vi "ProjectDataTransToStringForLog.vi"(7 "Class Name":string, 9 "NewVal":variant, 10 "OldVal":variant, 11 "Label.Text":string) -> (1 "NewData":string, 2 "OldData":string, 3 "DataName":string)   [LabVIEW 2019]
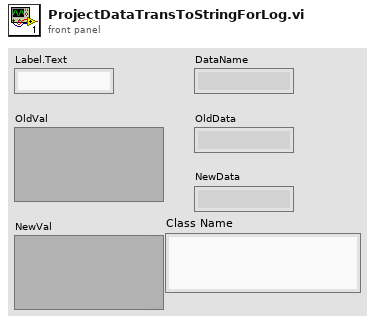
[diagram p1: front panel]
types:
  T1 = cluster{"Yield¢İvertake":dbl, "Fail¢İvertake":dbl, "TestTimeout":sgl, "TrayIn_Retry":dbl, "TrayOut_Retry":dbl, "Errcont":dbl, "back1":dbl, "back2":dbl}
  T2 = cluster{"Yield¢İvertake":dbl, "Fail¢İvertake":dbl, "TestTimeout":dbl, "TrayIn_Retry":dbl, "TrayOut_Retry":dbl, "Errcont":dbl, "back1":dbl, "back2":dbl}
  T3 = cluster{"PC-ID":string, "StationAddress":string}[]
  T4 = cluster{"SHB1":string, "SHB2":string, "SHB3":string, "SHB4":string, "SHB5":string, "SHB6":string, "SHB7":string, "SHB8":string}
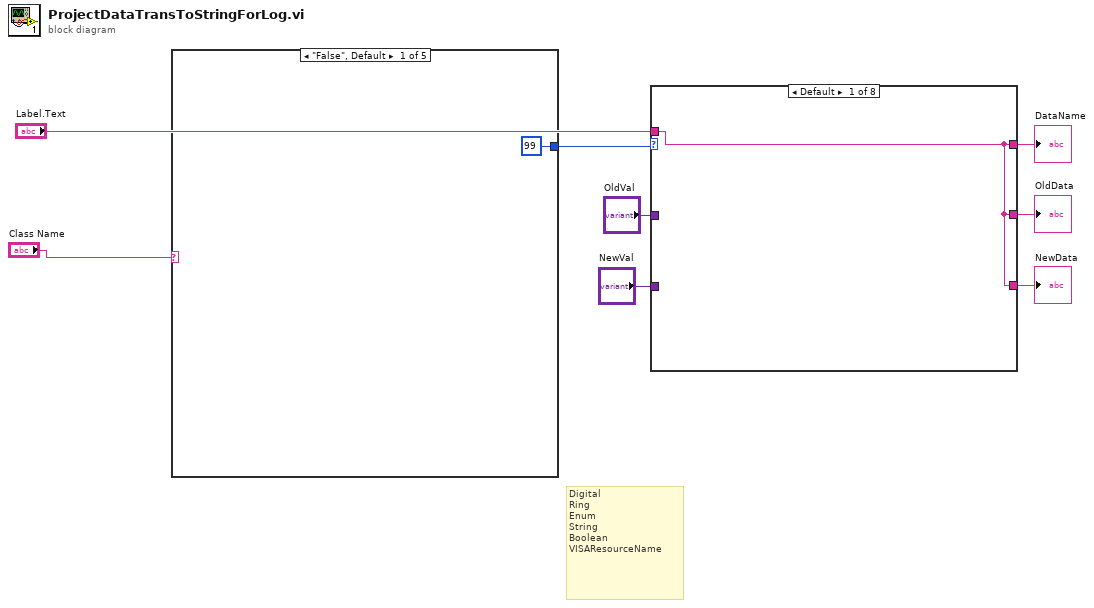
[diagram p0: block diagram]
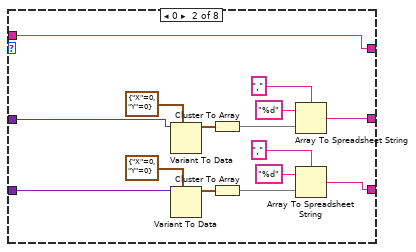
[diagram p2: hidden frame]
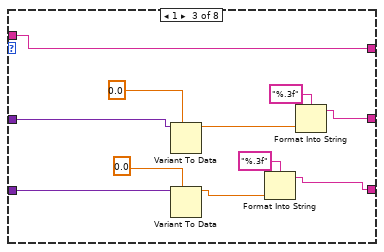
[diagram p3: hidden frame]
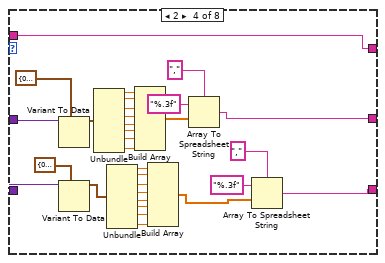
[diagram p4: hidden frame]
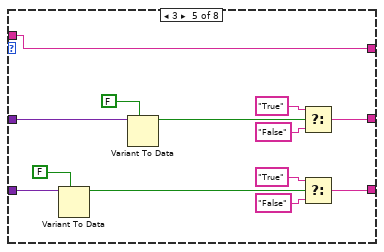
[diagram p5: hidden frame]
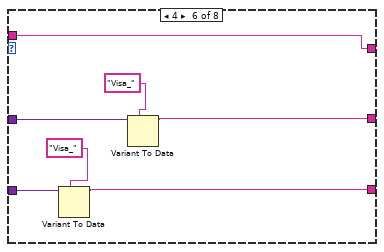
[diagram p6: hidden frame]
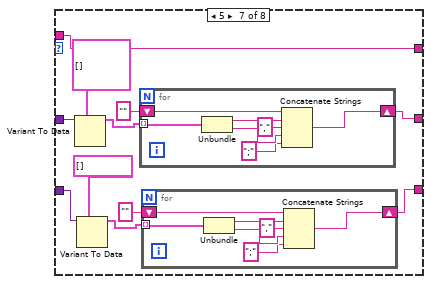
[diagram p7: hidden frame]
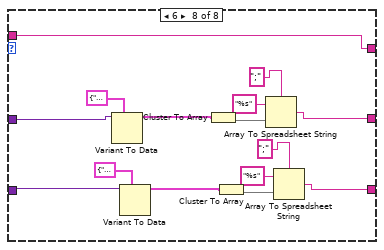
[diagram p8: hidden frame]
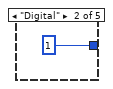
[diagram p9: hidden frame]
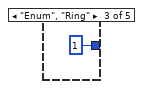
[diagram p10: hidden frame]
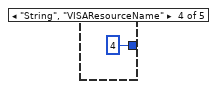
[diagram p11: hidden frame]
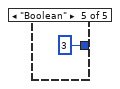
[diagram p12: hidden frame]
diagram:
  # "Digital\nRing\nEnum\nString\nBoolean\nVISAResourceName"
  n1 = case shown="\"False\", Default" "Class Name" {
    tunnel: [99 1 1 4 3] -> w1
    frame "False", Default {
    }
    frame "Digital" {
    }
    frame "Enum", "Ring" {
    }
    frame "String", "VISAResourceName" {
    }
    frame "Boolean" {
    }
  }
  n2 = case shown="Default" w1 {
    tunnel: "OldVal" -> [_ w29 w40 w68 w81 w90 w99 w119]
    tunnel: "NewVal" -> [_ w27 w39 w67 w84 w91 w93 w127]
    tunnel: [w14 w15 w30 w69 w72 w85 w101 w117] -> w4
    tunnel: [w14 w17 w31 w45 w74 w87 w100 w118] -> w5
    tunnel: [w14 w16 w32 w41 w73 w86 w92 w126] -> w6
    tunnel: "Label.Text" -> [w14 w15 w30 w69 w72 w85 w101 w117]
    frame Default {
    }
    frame 0 {
      n3 = Variant To Data(type=cluster{"X":i32, "Y":i32} {"X"=0, "Y"=0} ("DutTray"), Variant=w29) -> (data=w25:cluster{"X":i32, "Y":i32})  [unwired: 1 in, 1 out]
      n4 = Variant To Data(type=cluster{"X":i32, "Y":i32} {"X"=0, "Y"=0} ("DutTray"), Variant=w27) -> (data=w18:cluster{"X":i32, "Y":i32})  [unwired: 1 in, 1 out]
      n5 = Cluster To Array(cluster=w25) -> (array=w24:i32[])
      n6 = Cluster To Array(cluster=w18) -> (array=w19:i32[])
      n7 = Array To Spreadsheet String(delimiter (Tab)=",", array=w24, 3:"%d" ("format string")) -> (spreadsheet string=w17:string)
      n8 = Array To Spreadsheet String(delimiter (Tab)=",", array=w19, 3:"%d" ("format string")) -> (spreadsheet string=w16:string)
    }
    frame 1 {
      n9 = Variant To Data(type=0.0, Variant=w40) -> (data=w35:dbl)  [unwired: 1 in, 1 out]
      n10 = Variant To Data(type=0.0, Variant=w39) -> (data=w33:dbl)  [unwired: 1 in, 1 out]
      n11 = Format Into String(format string="%.3f", w33) -> (resulting string=w32:string)  [unwired: 2 in, 1 out]
      n12 = Format Into String(format string="%.3f", w35) -> (resulting string=w31:string)  [unwired: 2 in, 1 out]
    }
    frame 2 {
      n13 = Variant To Data(type=T2 {"Yield¢İvertake"=0.0, "Fail¢İvertake"=0.0, "TestTimeout"=0.0, "TrayIn_Retry"=3.0, "TrayOut_Retry"=0.0, "Errcont"=0.0, "back1"=0.0, "back2"=0.0} ("Res_Restrictions"), Variant=w68) -> (data=w66:T2)  [unwired: 1 in, 1 out]
      n14 = Variant To Data(type=T1 {"Yield¢İvertake"=0.0, "Fail¢İvertake"=0.0, "TestTimeout"=0.0, "TrayIn_Retry"=3.0, "TrayOut_Retry"=0.0, "Errcont"=0.0, "back1"=0.0, "back2"=0.0} ("Res_Restrictions"), Variant=w67) -> (data=w49:T1)  [unwired: 1 in, 1 out]
      n15 = Unbundle(w66) -> ("Yield¢İvertake"=w65:dbl, "Fail¢İvertake"=w64:dbl, "TestTimeout"=w63:dbl, "TrayIn_Retry"=w62:dbl, "TrayOut_Retry"=w61:dbl, "Errcont"=w60:dbl, "back1"=w59:dbl, "back2"=w58:dbl)
      n16 = Unbundle(w49) -> ("Yield¢İvertake"=w50:dbl, "Fail¢İvertake"=w51:dbl, "TestTimeout"=w52:sgl, "TrayIn_Retry"=w53:dbl, "TrayOut_Retry"=w54:dbl, "Errcont"=w55:dbl, "back1"=w56:dbl, "back2"=w57:dbl)
      n17 = Build Array(w65, w64, w63, w62, w61, w60, w59, w58) -> (w48:dbl[])
      n18 = Build Array(w50, w51, w52, w53, w54, w55, w56, w57) -> (w42:dbl[])
      n19 = Array To Spreadsheet String(delimiter (Tab)=",", array=w48, 3:"%.3f" ("format string")) -> (spreadsheet string=w45:string)
      n20 = Array To Spreadsheet String(delimiter (Tab)=",", array=w42, 3:"%.3f" ("format string")) -> (spreadsheet string=w41:string)
    }
    frame 3 {
      n21 = Variant To Data(type=FALSE ("linkSFCS"), Variant=w84) -> (data=w75:bool)  [unwired: 1 in, 1 out]
      n22 = Variant To Data(type=FALSE ("linkSFCS"), Variant=w81) -> (data=w80:bool)  [unwired: 1 in, 1 out]
      n23 = Select(t="True", s=w80, f="False") -> (s? t:f=w74:string)
      n24 = Select(t="True", s=w75, f="False") -> (s? t:f=w73:string)
    }
    frame 4 {
      n25 = Variant To Data(type="Visa_" ("regular expression"), Variant=w91) -> (data=w86:string)  [unwired: 1 in, 1 out]
      n26 = Variant To Data(type="Visa_" ("regular expression"), Variant=w90) -> (data=w87:string)  [unwired: 1 in, 1 out]
    }
    frame 5 {
      n27 = Variant To Data(type=T3 [] ("Define_Station"), Variant=w99) -> (data=w97:T3)  [unwired: 1 in, 1 out]
      n28 = Variant To Data(type=T3 [] ("Define_Station"), Variant=w93) -> (data=w96:T3)  [unwired: 1 in, 1 out]
      n29 = for {
        tunnel: w97 -> [w116] mode=indexing
        shift-right: [w111] -> w100
        shift-left: "" -> [w110]
        n30 = Unbundle(w116) -> ("PC-ID"=w115:string, "StationAddress"=w113:string)
        n31 = Concatenate Strings(w110, w115, "," ("string"), w113, ";" ("string")) -> (w111:string)
      }
      n32 = for {
        tunnel: w96 -> [w109] mode=indexing
        shift-right: [w104] -> w92
        shift-left: "" -> [w103]
        n33 = Unbundle(w109) -> ("PC-ID"=w108:string, "StationAddress"=w106:string)
        n34 = Concatenate Strings(w103, w108, "," ("string"), w106, ";" ("string")) -> (w104:string)
      }
    }
    frame 6 {
      n35 = Variant To Data(type=T4 {"SHB1"="", "SHB2"="", "SHB3"="", "SHB4"="", "SHB5"="", "SHB6"="", "SHB7"="", "SHB8"=""} ("8SData_VisionRef"), Variant=w119) -> (data=w123:T4)  [unwired: 1 in, 1 out]
      n36 = Variant To Data(type=T4 {"SHB1"="", "SHB2"="", "SHB3"="", "SHB4"="", "SHB5"="", "SHB6"="", "SHB7"="", "SHB8"=""} ("8SData_VisionRef"), Variant=w127) -> (data=w128:T4)  [unwired: 1 in, 1 out]
      n37 = Cluster To Array(cluster=w123) -> (array=w122:string[])
      n38 = Cluster To Array(cluster=w128) -> (array=w129:string[])
      n39 = Array To Spreadsheet String(delimiter (Tab)=";", array=w122, 3:"%s" ("format string")) -> (spreadsheet string=w118:string)
      n40 = Array To Spreadsheet String(delimiter (Tab)=";", array=w129, 3:"%s" ("format string")) -> (spreadsheet string=w126:string)
    }
  }
  "NewData" <- w6
  "OldData" <- w5
  "DataName" <- w4
